vi "APS jog start.vi"(8 "error in (no error)":errorcluster caption="错误输入（无错误）", 10 "On":i32, 11 "Axis_ID":i32) -> (0 "error out":errorcluster caption="错误输出", 3 "function return":i32)   [LabVIEW 2017, in "APS168.lvlib"]
doc: "I32 FNTYPE APS_jog_start( I32 Axis_ID, I32 On );"
uses:
  APS168.lvlib
  APS168.dll
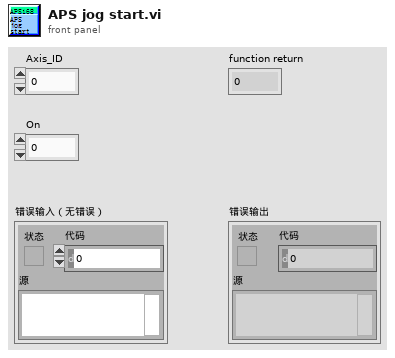
[diagram p1: front panel]
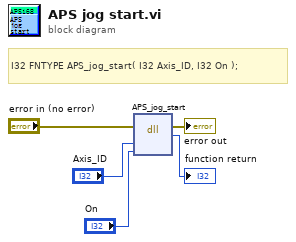
[diagram p0: block diagram]
diagram:
  # "I32 FNTYPE APS_jog_start( I32 Axis_ID, I32 On );"
  n1 = dll-call lib="PTH2Gabs E迈治LV范例testSubVIsADLINKMotion204cAPS168.*" fn="APS_jog_start"(error in="error in (no error)", "Axis_ID"="Axis_ID", "On"="On") -> (error out=→"error out":errorcluster, →"function return":i32)  [unwired: 4 in, 1 out]
